vi "Q.Enqueue Function.vi"(4 "RetSubCmd":string, 5 "Top of Q":bool, 6 "RetCmd (Default is 'TASK')":string="Task", 7 "Q Name":string, 8 "Error In":errorcluster, 9 "Data1":variant, 10 "Task Name":string, 11 "Q In":refnum<queue>) -> (0 "error out":errorcluster, 2 "SeqNum":i32, 3 "Q Out":refnum<queue>)   [LabVIEW 2024, in "EQMF.lvlib" / "Queue Utils.lvlib"]
doc: "This VI enqueues a Task:\n Queue element 'Cmd' = \"Task\"\n Queue element 'Sub' is assigned to the value of the 'Task Name' input.\n\nThis VI obtains the queue by name or by queue reference.\nIf the 'Q Name' input is empty then it obtains the queue by the 'Q In\" reference.\nIf the 'Q Name' input is NOT empty then it obtains the queue by the this name.\n If a queue is ontained by name and the queue does not already exits, an error is generated.\n\nThe 'Top of Q' input is FALSE by default.\nThis input will cause this item to be enqueued on the top of the queue when it is TRUE."
uses:
  Queue Utils.lvlib
  Q.Element.ctl
  Q.Msg Return Info.ctl
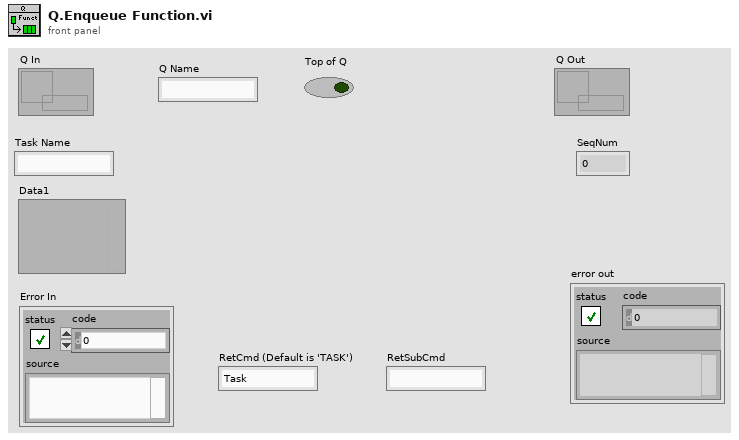
[diagram p1: front panel]
types:
  T1 = typedef "EQMF.lvlib/Queue Utils.lvlib/Q.Msg Return Info.ctl" = cluster{"Ret Q":refnum<queue>, "Ret Msg":T2, "SeqNum":i32}
  T2 = typedef "EQMF.lvlib/Queue Utils.lvlib/Q.Element.ctl" = cluster{"Cmd":string, "Sub":string, "Data1":variant, "Data2":variant}
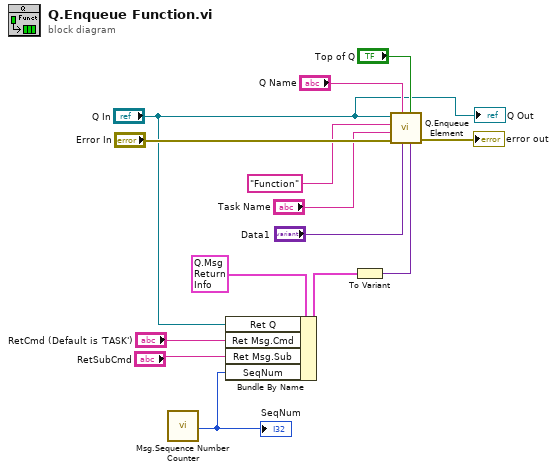
[diagram p0: block diagram]
diagram:
  n1 = call "Msg.Sequence Number Counter.vi"() -> ("SeqNum"=w2:i32)  [unwired: 1 in]
  "SeqNum" <- w2
  n2 = Bundle By Name(cluster=T1 {"Ret Q"=refnum, "Ret Msg"={"Cmd"="", "Sub"="", "Data1"=variant, "Data2"=variant}, "SeqNum"=0} ("Cmd Ret Req Data"), "Ret Q"="Q In", "Ret Msg.Cmd"="RetCmd (Default is 'TASK')", "Ret Msg.Sub"="RetSubCmd", "SeqNum"=w2) -> (w6:T1)
  n3 = To Variant(anything=w6) -> (Variant=w5:variant)
  n4 = call "Q.Enqueue Element.vi"("Data2"=w5, "Top of Q"="Top of Q", "Data1"="Data1", "Q Name"="Q Name", "error in"="Error In", "Sub"="Task Name", "Cmd"="Function", "Q In"="Q In") -> ("error out"=→"error out":errorcluster)  [unwired: 2 in, 1 out]
  "Q Out" <- "Q In"
